vi "Yokogawa WT1800 Series Measure Normal.vi"() -> ()   [LabVIEW 2015]
doc: "This example shows how to use ranging configuration and measure the normal numeric data."
uses:
  <instrlib>/Yokogawa WT1800 Series/Public/Utility/Function/Create Function String (Voltage).vi
  <instrlib>/Yokogawa WT1800 Series/Public/Data/Low Level/Fetch Measurement (Normal).vi
  <instrlib>/Yokogawa WT1800 Series/Yokogawa WT1800 Series.lvlib
panel:
  in  "Element/Wiring Unit (1: 1)":i32(ring)=1 items=["1"=1, "2"=2, "3"=3, "4"=4, "5"=5, "6"=6, "Sigma A"=7, "Sigma B"=8, "Sigma C"=9]
  in  "Function (0: Urms)":i32(ring) items=["Urms", "Umn", "Udc", "Urmn", "Uac", "U+peak", "U-peak", "CfU"]
  out "Function":string
  out "Measurement":dbl
  in  "Item (1)":i32=1 min=1 max=255 step=1
  in  "Timeout (10000 ms)":i32=10000 min=1
  in  "VISA resource name":refnum<visa-resource-name>
  # "(c) 2011 Yokogawa Meters & Instruments Corporation.  All rights reserved."
  # "WT1800 SERIES POWER ANALYZER"
  # "ms"
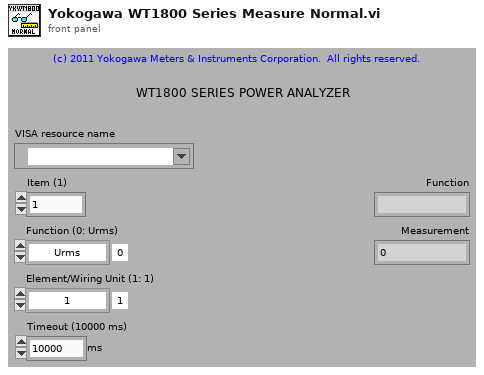
[diagram p1: front panel]
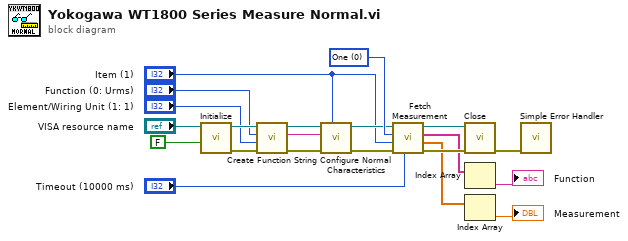
[diagram p0: block diagram]
diagram:
  w16 = 0 items=["One", "Plural"] ("Measure Item (1: Plural)")
  n1 = call <instrlib>:"Initialize.vi"("Reset (True)"=FALSE ("Reset? (True)"), "VISA resource name"="VISA resource name") -> ("error out"=w12:errorcluster, "VISA resource name out"=w13:refnum<visa-resource-name>)  [unwired: 8 in]
  n2 = call-poly <instrlib>:"Create Function String.vi"("error in (no error)"=w12, "Element/Wiring Unit (1: 1)"="Element/Wiring Unit (1: 1)", "Function (0: Urms)"="Function (0: Urms)", "VISA resource name"=w13) -> ("error out"=w10:errorcluster, "Function String"=w1:string, "VISA resource name out"=w11:refnum<visa-resource-name>)  [unwired: 5 in]
  n3 = call <instrlib>:"Configure Normal Characteristics.vi"("Item (1)"="Item (1)", "error in (no error)"=w10, "Function (Empty)"=w1, "VISA resource name"=w11) -> ("error out"=w14:errorcluster, "VISA resource name out"=w15:refnum<visa-resource-name>)  [unwired: 6 in]
  n4 = call-poly <instrlib>:"Fetch Measurement.vi"("Timeout (10000 ms)"="Timeout (10000 ms)", "error in (no error)"=w14, "Number of Item (15)"="Item (1)", "Measure Item (1: Plural)"=w16, "VISA resource name"=w15) -> ("error out"=w18:errorcluster, "Measurement"=w9:dbl[], "Function"=w5:string[], "VISA resource name out"=w19:refnum<visa-resource-name>)  [unwired: 3 in]
  n5 = call <instrlib>:"Close.vi"("error in (no error)"=w18, "VISA resource name"=w19) -> ("error out"=w21:errorcluster)  [unwired: 9 in]
  n6 = Index Array(array=w5) -> (element=→"Function":string)  [unwired: 1 in]
  n7 = Index Array(array=w9) -> (element=→"Measurement":dbl)  [unwired: 1 in]
  n8 = call <vilib>:"Simple Error Handler.vi"("error in (no error)"=w21) -> ()  [unwired: 4 in, 5 out]
